vi "mspec stitcher get images.vi"(11 "Stitcher in":refnum<class "MagSpecStitcher.lvclass">) -> (1 "Timed out":bool, 2 "variant out":variant, 3 "MagSpecStitcher.lvclass 2":refnum<class "MagSpecStitcher.lvclass">, 4 "OK":bool[](array[boolean]))   [LabVIEW 2020, in "MagSpecStitcher.lvclass"]
uses:
  MagSpecStitcher.lvclass
  C:/GEECS/Developers Version/source/Device Drivers/BaseDriver/BaseDriver.lvclass
  MagSpecStitcher.lvclass/MagSpecStitcher.ctl
  BaseDriver/BaseDriver.lvclass
panel:
  out "Shotnumbers 2":i32[][](array[numeric])
  out "Shotnumbers":i32[](array[numeric])
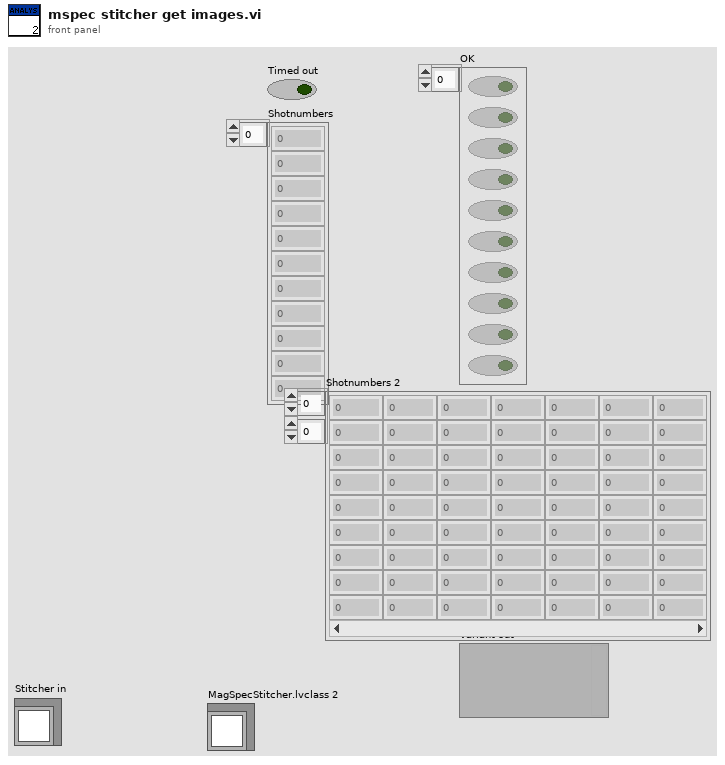
[diagram p1: front panel]
types:
  T1 = typedef "SubscriberCluster_TypDEf.ctl" = cluster{"tcp data event":T2, "Event Registration Refnum":refnum<event-registration>, "data queue":refnum<queue>, "Devices":string[], "Alias":string[], "Variable header":string[], "Devices ALL":string[]}
  T2 = typedef "tcp_new_data_event.ctl" = refnum<user-event>
  T3 = typedef "MagSpecStitcher.lvclass/analysis_data_typdef.ctl" = cluster{"MagSpecA":T4, "MagSpecB":T4, "MagSpecC":T4, "MagSpecD":T4, "MagSpecG":T4, "MagSpecH":T4, "MagSpecI":T4, "MagSpecJ":T4, "MagSpecK":T4, "MagSpecL":T4, "EnergyAxisA":dbl[], "AngleAxisA":dbl[], "EnergyAxisB":dbl[], "AngleAxisB":dbl[], "EnergyAxisC":dbl[], "AngleAxisC":dbl[], "EnergyAxisD":dbl[], "AngleAxisD":dbl[], "EnergyAxisG":dbl[], "AngleAxisG":dbl[], "EnergyAxisH":dbl[], "AngleAxisH":dbl[], "EnergyAxisI":dbl[], "AngleAxisI":dbl[], "EnergyAxisJ":dbl[], "AngleAxisJ":dbl[], "EnergyAxisK":dbl[], "AngleAxisK":dbl[], "EnergyAxisL":dbl[], "AngleAxisL":dbl[], "MaxPicoCoulombA":dbl, "MaxPicoCoulombB":dbl, "MaxPicoCoulombC":dbl, "MaxPicoCoulombD":dbl, "MaxPicoCoulombG":dbl, "MaxPicoCoulombH":dbl, "MaxPicoCoulombI":dbl, "MaxPicoCoulombJ":dbl, "MaxPicoCoulombK":dbl, "MaxPicoCoulombL":dbl, "acqtimestamp":dbl}
  T4 = typedef "IMAQ Image.ctl" = refnum<image>
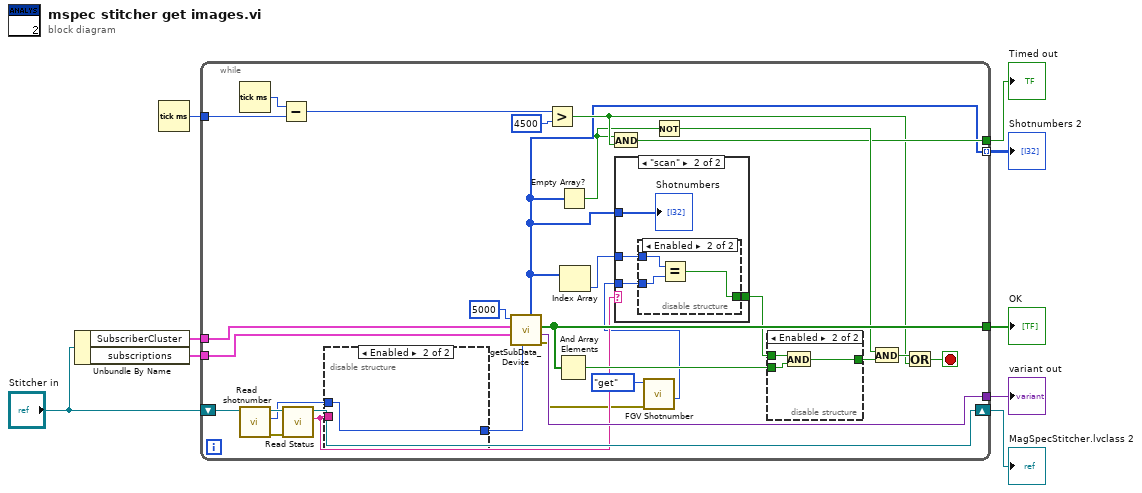
[diagram p0: block diagram]
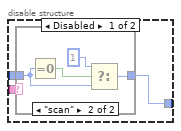
[diagram p2: hidden frame]
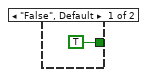
[diagram p4: hidden frame]
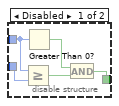
[diagram p5: hidden frame]
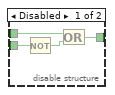
[diagram p6: hidden frame]
diagram:
  n1 = Unbundle By Name("Stitcher in") -> ("SubscriberCluster"=w4:T1, "subscriptions"=w3:T3)
  n2 = Tick Count (ms)() -> (millisecond timer value=w8:u32)
  n3 = while {
    tunnel: w4 -> [w39]
    tunnel: [w22] -> w7
    tunnel: [w36] -> w6
    tunnel: w3 -> [w21]
    tunnel: w8 -> [w32]
    tunnel: [w25] -> w9
    tunnel: [w20] -> w5 mode=indexing
    shift-right: [w18] -> w1
    shift-left: "Stitcher in" -> [w17]
    stop <- w29 stop-if-true
    n4 = Tick Count (ms)() -> (millisecond timer value=w33:u32)
    n5 = call-dynamic "Read shotnumber.vi"("BaseDriver in"=w17) -> ("error out"=w19:errorcluster, "shotnumber"=w14:i32, "BaseDriver out"=w16:refnum<class "MagSpecStitcher.lvclass">)  [unwired: 7 in, 1 out]
    n6 = Subtract(x=w33, y=w32) -> (x-y=w31:u32)
    n7 = call "Read Status.vi"("error in (no error)"=w19, "BaseDriver in"=w16) -> ("Status"=w15:string, "BaseDriver out"=w18:refnum<class "MagSpecStitcher.lvclass">)  [unwired: 7 in, 1 out]
    n8 = disable-structure shown="Enabled" {
      disable-tunnel: w15 -> [w42 _]
      disable-tunnel: w14 -> [w41 w48]
      disable-tunnel: [w40 w48] -> w13
      frame Disabled {
        n9 = case shown="\"scan\"" w42 {
          tunnel: w41 -> [w43 w46]
          tunnel: [w43 w44] -> w40
          frame "False", Default {
          }
          frame "scan" {
            n10 = Equal To 0?(x=w46) -> (x = 0?=w47:bool)
            n11 = Select(t=1, s=w47, f=w46) -> (s? t:f=w44:i32)
          }
        }
      }
      frame Enabled {
      }
    }
    n12 = call "getSubData_Device.vi"("shotnumber"=w13, "variant in"=w21, "SubscriberCluster"=w39, "timeout"=5000) -> ("error out"=w11:errorcluster, "variant out"=w22:variant, "OK"=w36:bool[], "Shotnumbers"=w20:i32[])  [unwired: 3 in, 1 out]
    n13 = Greater?(x=w31, y=u32 4500) -> (0:w24:bool)
    n14 = And Array Elements(Boolean array=w36) -> (logical AND=w35:bool)
    n15 = Empty Array?(array=w20) -> (empty?=w23:bool)
    n16 = Index Array(array=w20) -> (element=w37:i32)  [unwired: 1 in]
    n17 = And(x=w23, y=w24) -> (x .and. y?=w25:bool)
    n18 = call "FGV Shotnumber.vi"("error in (no error)"=w11, "command"=enum16{"set", "get", "reset"}."get") -> ("shot#"=w10:i32)  [unwired: 7 in, 2 out]
    n19 = case shown="\"scan\"" w15 {
      tunnel: w37 -> [_ w52]
      tunnel: w10 -> [_ w51]
      tunnel: [TRUE w53] -> w34
      tunnel: w20 -> [_ w50]
      frame "False", Default {
      }
      frame "scan" {
        n20 = disable-structure shown="Enabled" {
          disable-tunnel: [w57 w59] -> w53
          disable-tunnel: w52 -> [w56 w60]
          disable-tunnel: w51 -> [w55 w61]
          frame Disabled {
            n21 = Greater Or Equal?(x=w56, y=w55) -> (x >= y?=w54:bool)
            n22 = Greater Than 0?(x=w56) -> (x > 0?=w58:bool)
            n23 = And(x=w58, y=w54) -> (x .and. y?=w57:bool)
          }
          frame Enabled {
            n24 = Equal?(x=w60, y=w61) -> (x = y?=w59:bool)
          }
        }
        "Shotnumbers" <- w50
      }
    }
    n25 = Not(x=w23) -> (.not. x?=w28:bool)
    n26 = disable-structure shown="Enabled" {
      disable-tunnel: w35 -> [w65 w67]
      disable-tunnel: [w64 w66] -> w27
      disable-tunnel: w34 -> [w63 w68]
      frame Disabled {
        n27 = Not(x=w65) -> (.not. x?=w62:bool)
        n28 = Or(x=w63, y=w62) -> (x .or. y?=w64:bool)
      }
      frame Enabled {
        n29 = And(x=w68, y=w67) -> (x .and. y?=w66:bool)
      }
    }
    n30 = And(x=w28, y=w27) -> (x .and. y?=w26:bool)
    n31 = Or(x=w26, y=w24) -> (x .or. y?=w29:bool)
  }
  "Timed out" <- w9
  "variant out" <- w7
  "OK" <- w6
  "Shotnumbers 2" <- w5
  "MagSpecStitcher.lvclass 2" <- w1
